vi "Memory.Pointer.Read.Safe.0D.I8.vi"(8 "error in (no error)":errorcluster, 10 "value in":i8, 11 "pointer in":refnum<class "Memory.Pointer.lvclass">) -> (0 "error out":errorcluster, 2 "value out":i8, 3 "pointer out":refnum<class "Memory.Pointer.lvclass">)   [LabVIEW 2016, in "Memory Manager.lvlib" / "Memory.Pointer.lvclass"]
doc: "Reads the contents of the address specified by <b>pointer</b> into <b>value</b>.\n\n<b>Note:</b> This VI is <b>safe</b>.\n\nSafe means that this function evaluates the size parameter of <b>pointer</b> to ensure that is inbounds of allocated memory before peforming a memory read/write. Reading/writing more data to a pointer than it has allocated can corrupt or crash LabVIEW."
uses:
  Memory.Pointer.lvclass
  Memory.Pointer.lvclass/Memory.Pointer.ctl
  Accessors/Get Address.vi
  Memory.Pointer.Errors.vi
  Memory.Pointer.Errors.Out of Bounds.vi
  Accessors/Get Size.vi
  Submodules/Static Error Handling/Source/Library/VIs/Static Error Handling.Source Buffer.Write.String.vi
  Memory.Pointer.Errors.Write Pointer Size.vi
  Memory.Pointer.Errors.Create Error.vi
  Submodules/Static Error Handling/Source/Library/VIs/Static Error Handling.Source Buffer.Write.Numeric.Scalar.Base10.vi
  Submodules/Static Error Handling/Source/Library/VIs/Static Error Handling.Source Buffer.Write.Numeric.Scalar.Base10 (U64).vi
  Submodules/Static Error Handling/Source/Library/VIs/Static Error Handling.Error Cluster Constant.vi
  Submodules/Static Error Handling/Source/Library/VIs/Static Error Handling.Error Cluster Constant (256B).vi
  Submodules/Static Error Handling/Source/Library/VIs/Static Error Handling.Parameters.Status.Set.vi
  Submodules/Static Error Handling/Source/Library/VIs/Static Error Handling.Parameters.Code.Set.vi
  Submodules/Static Error Handling/Source/Library/VIs/Static Error Handling.Parameters.VI Source.Set.vi
  Constants/Memory.Constants.vi
  Constants/Memory.Constants.Library Name.vi
  Memory.Pointer.Errors.Get Info.vi
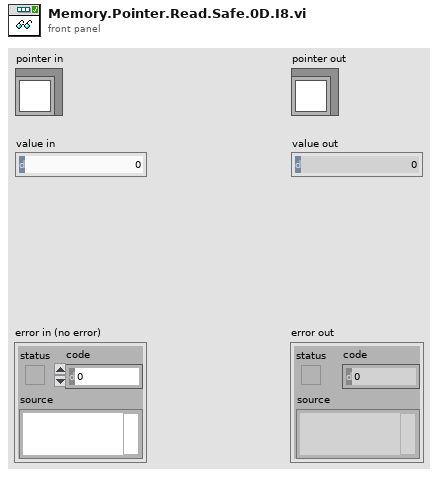
[diagram p1: front panel]
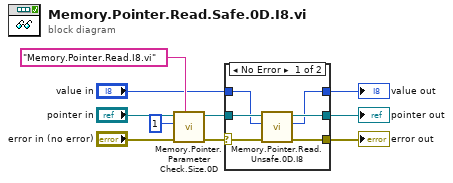
[diagram p0: block diagram]
diagram:
  n1 = call "Memory.Pointer.Parameter Check.Size.0D.vi"("source vi name"="Memory.Pointer.Read.I8.vi", "error in (no error)"="error in (no error)", "required size"=u64 1 ("y"), "Pointer in"="pointer in") -> ("error out"=w8:errorcluster, "Pointer out"=w10:refnum<class "Memory.Pointer.lvclass">)  [unwired: 5 in, 1 out]
  n2 = case shown="No Error" w8 {
    selector: w8 -> [w12 w17]
    tunnel: w10 -> [w16 w19]
    tunnel: [w15 w19] -> w3
    tunnel: [w14 w18] -> w5
    tunnel: "value in" -> [w13 w18]
    tunnel: [w11 w17] -> w2
    frame No Error {
      n3 = call "Memory.Pointer.Read.Unsafe.0D.I8.vi"("error in (no error)"=w12, "value in"=w13, "pointer in"=w16) -> ("error out"=w11:errorcluster, "value out"=w14:i8, "pointer out"=w15:refnum<class "Memory.Pointer.lvclass">)  [unwired: 6 in]
    }
    frame Error {
    }
  }
  "error out" <- w2
  "pointer out" <- w3
  "value out" <- w5
